vi "send abs move to stage.vi"(8 "error in (no error)":errorcluster, 9 "absolute focus position":dbl[unit], 10 "absolute z position":dbl[unit], 11 "Autofocus in":refnum<class "Autofocus.lvclass">) -> (0 "error out":errorcluster, 3 "Autofocus out":refnum<class "Autofocus.lvclass">)   [LabVIEW 2012, in "Autofocus.lvclass"]
uses:
  Autofocus.lvclass
  <vilib>/Distrio/Murmex/GenericMessage/GenericMessage.lvclass
  <vilib>/Distrio/Murmex/StartMessage/StartMessage.lvclass
  Autofocus.lvclass/Autofocus.ctl
  <vilib>/Distrio/Murmex/Message/Message.lvclass
  <vilib>/Distrio/Murmex/Murmex/Murmex.lvclass
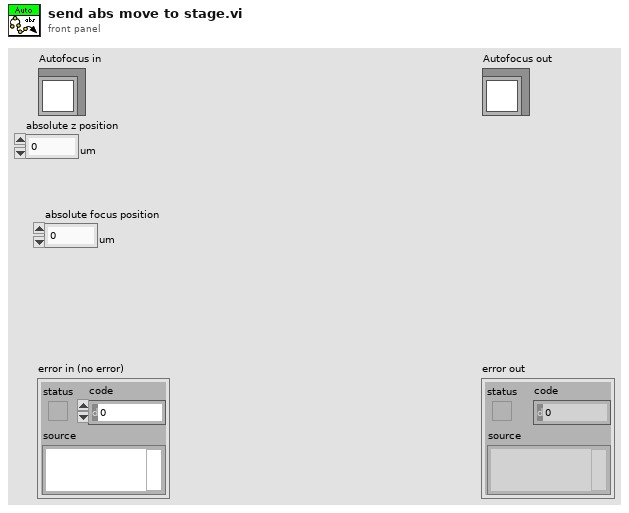
[diagram p1: front panel]
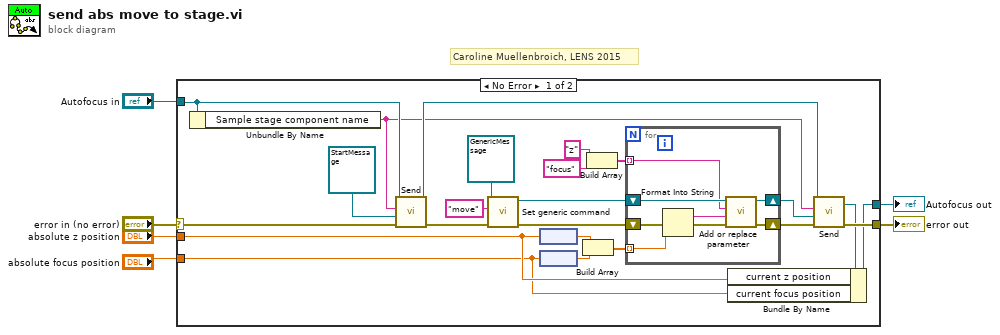
[diagram p0: block diagram]
diagram:
  # "Caroline Muellenbroich, LENS 2015"
  n1 = case shown="No Error" "error in (no error)" {
    selector: "error in (no error)" -> [w19 w39]
    tunnel: [w23 w39] -> w5
    tunnel: [w21 w38] -> w3
    tunnel: "Autofocus in" -> [w17 w38]
    tunnel: "absolute z position" -> [w20 _]
    tunnel: "absolute focus position" -> [w13 _]
    frame No Error {
      n2 = Unbundle By Name(w17) -> ("Sample stage component name"=w15:string)
      n3 = call <vilib>:"Send.vi"("error in (no error)"=w19, "Message"=refnum<class "StartMessage.lvclass"> refnum ("Message in"), "recipient"=w15, "Murmex in"=w17) -> ("error out"=w18:errorcluster, "Murmex out"=w16:refnum<class "Autofocus.lvclass">)  [unwired: 6 in]
      n4 = call <vilib>:"Set generic command.vi"("error in (no error)"=w18, "generic command"="move" ("command string"), "GenericMessage in"=refnum<class "GenericMessage.lvclass"> refnum ("Murmex.lvlib:GenericMessage")) -> ("error out"=w25:errorcluster, "GenericMessage out"=w24:refnum<class "GenericMessage.lvclass">)  [unwired: 7 in]
      n5 = node(w20) -> (w9:dbl)
      n6 = node(w13) -> (w8:dbl)
      n7 = Build Array(w9, w8) -> (w7:dbl[])
      n8 = Build Array("z" ("name"), "focus" ("name")) -> (w10:string[])
      n9 = for {
        tunnel: w7 -> [w31] mode=indexing
        shift-right: [w37] -> w29
        shift-left: w24 -> [w32]
        shift-right: [w36] -> w28
        shift-left: w25 -> [w33]
        tunnel: w10 -> [w30] mode=indexing
        n10 = Format Into String(error in=w33, w31) -> (resulting string=w35:string, error out=w34:errorcluster)  [unwired: 2 in]
        n11 = call <vilib>:"Add or replace parameter.vi"("error in (no error)"=w34, "value"=w35, "name"=w30, "Message in"=w32) -> ("error out"=w36:errorcluster, "Message out"=w37:refnum<class "GenericMessage.lvclass">)  [unwired: 6 in]
      }
      n12 = call <vilib>:"Send.vi"("error in (no error)"=w28, "Message"=w29, "recipient"=w15, "Murmex in"=w16) -> ("error out"=w23:errorcluster, "Murmex out"=w22:refnum<class "Autofocus.lvclass">)  [unwired: 6 in]
      n13 = Bundle By Name(cluster=w22, "current z position"=w20, "current focus position"=w13) -> (w21:refnum<class "Autofocus.lvclass">)
    }
    frame Error {
    }
  }
  "error out" <- w5
  "Autofocus out" <- w3
